vi "ChangeAverage.vi"(8 "Averages":i32, 9 "error in (no error)":errorcluster, 11 "VISA resource name":refnum<visa-resource-name>) -> (0 "error out":errorcluster)   [LabVIEW 2023, in "KeysightN9020B.lvlib"]
uses:
  KeysightN9020B.lvlib
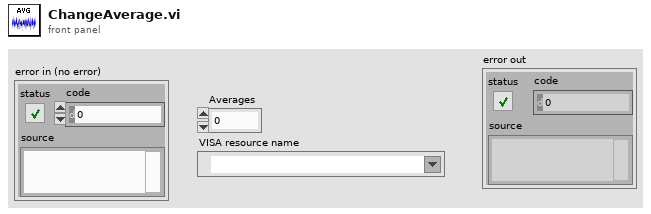
[diagram p1: front panel]
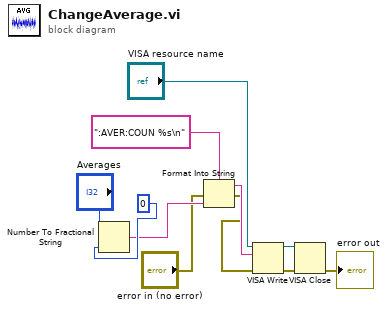
[diagram p0: block diagram]
diagram:
  n1 = Number To Fractional String(number="Averages", precision (6)=i16 0) -> (F-format string=w5:string)  [unwired: 2 in]
  n2 = Format Into String(format string=":AVER:COUN %s\n" ("string"), error in="error in (no error)", w5) -> (resulting string=w4:string, error out=w1:errorcluster)  [unwired: 1 in]
  n3 = VISA Write(VISA resource name="VISA resource name", write buffer=w4, error in (no error)=w1) -> (VISA resource name out=w8:refnum<visa-resource-name>, error out=w10:errorcluster)  [unwired: 1 out]
  n4 = VISA Close(VISA resource name=w8, error in (no error)=w10) -> (error out=→"error out":errorcluster)
